vi "example_2_6_a.vi"() -> ()   [LabVIEW 2018]
panel:
  out "Numeric Indicator":i16
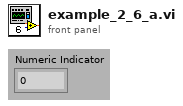
[diagram p1: front panel]
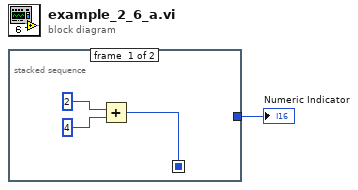
[diagram p0: block diagram]
diagram:
  n1 = stacked-sequence {
    seq-local: [w2 _] -> [_ w5]
    tunnel: [_ w5] -> w1
    frame #0 {
      n2 = Add(x=2, y=4) -> (x+y=w2:i32)
    }
    frame #1 {
    }
  }
  "Numeric Indicator" <- w1
